vi "Main Editor UI.vi"() -> ()   [LabVIEW 2015, in "DAQmx Module editor node.lvclass"]
doc: "This is the main view for configuration the behavior of a module in the DCAF standard editor."
uses:
  DAQmx Module editor node.lvclass
  <vilib>/NI/Configuration Framework/Node/NodeRef.ctl
  <vilib>/NI/Configuration Framework/Node/NISE_CEF_Node.lvclass
  <vilib>/NI/AMC/Message Queue.ctl
  <vilib>/NI/AMC/Message.ctl
  <vilib>/NI/Tools/Keyed Array/KeyedArray.ctl
  <vilib>/NI/Configuration Framework/Node/UserEventRef.ctl
  <vilib>/NI/Configuration Framework/Controls/EventCluster.ctl
  <vilib>/NI/DCAF UI Toolkit/Controls/Configure.ctl
  <vilib>/NI/DCAF UI Toolkit/Controls/Add.ctl
  <vilib>/NI/DCAF UI Toolkit/Controls/Remove.ctl
  <vilib>/NI/Configuration Framework/Node/StopEvent.ctl
  <vilib>/NI/Configuration Framework/Node/RefreshUIEvent.ctl
  <vilib>/NI/Configuration Framework/Node/CacheState.ctl
  <vilib>/NI/Configuration Framework/Node/NodeChangeEvent.ctl
  <vilib>/NI/DCAF/Tag Editor Core/Table API/Available Tag Menu/channel action event.ctl
  <vilib>/NI/DCAF/Tag Editor Core/Table API/Available Tag Menu/dialog output action.ctl
  <vilib>/NI/Tag Bus Module Framework/channel/TBM channel.lvclass
  <vilib>/NI/Tag Bus/tag/tag descriptor.lvclass
  <vilib>/NI/DCAF/Tag Editor Core/Table API/Table Manager/Call Back Ref Type Def.ctl
  <vilib>/NI/DCAF/Tag Editor Core/Configuration Editor/Classes/Engine Parent/Engine Parent Editor Node.lvclass
  <vilib>/NI/DCAF/Tag Editor Core/Configuration Editor/Classes/Module editor node/module editor node.lvclass
  <vilib>/NI/DCAF UI Toolkit/Controls/Import.ctl
  <vilib>/NI/DCAF UI Toolkit/Controls/Export.ctl
  <vilib>/NI/DCAF/Tag Editor Core/Table API/Table Manager/references.ctl
  module/configuration/Daqmx Module configuration.lvclass/Daqmx Module configuration.ctl
  <vilib>/Utility/miscctls.llb/LVPositionTypeDef.ctl
  <vilib>/NI/DCAF/Tag Editor Core/Table API/Listbox/Multi Column Listbox.lvclass
  <vilib>/NI/Configuration Framework/NISE_CEF_TreeControl.lvlib
  <vilib>/NI/Tools/Keyed Array/Tools_KeyedArray.lvlib
  <vilib>/NI/AMC/AMC.lvlib
  <vilib>/NI/DCAF/Tag Editor Core/Table API/Table Manager.lvlib
  <vilib>/NI/DCAF/Tag Editor Core/Table API/Table Manager/Table Manager.lvclass
  <vilib>/NI/DCAF UI Toolkit/Controls/DCAF UI Elements.lvlib
  module/configuration/Daqmx Module configuration.lvclass
panel:
  in  "user event out":refnum<user-event>
  in  "node change":T1
  in  "cache state":T2
  in  "refresh UI":T3
  in  "stop event":T4
  in  "Tab Control":T5(tab)
  in  "Remove Button":T6
  in  "Add Button":T7
  in  "Table":i32(listbox)
  in  "settings":T8
  in  "Export":T9
  in  "Import":T10
  in  "Data Rate (Hz)":dbl=1.0 min=1.0 step=1.0
  in  "user event":T11
  in  "main queue":T12
  in  "node ref":T13
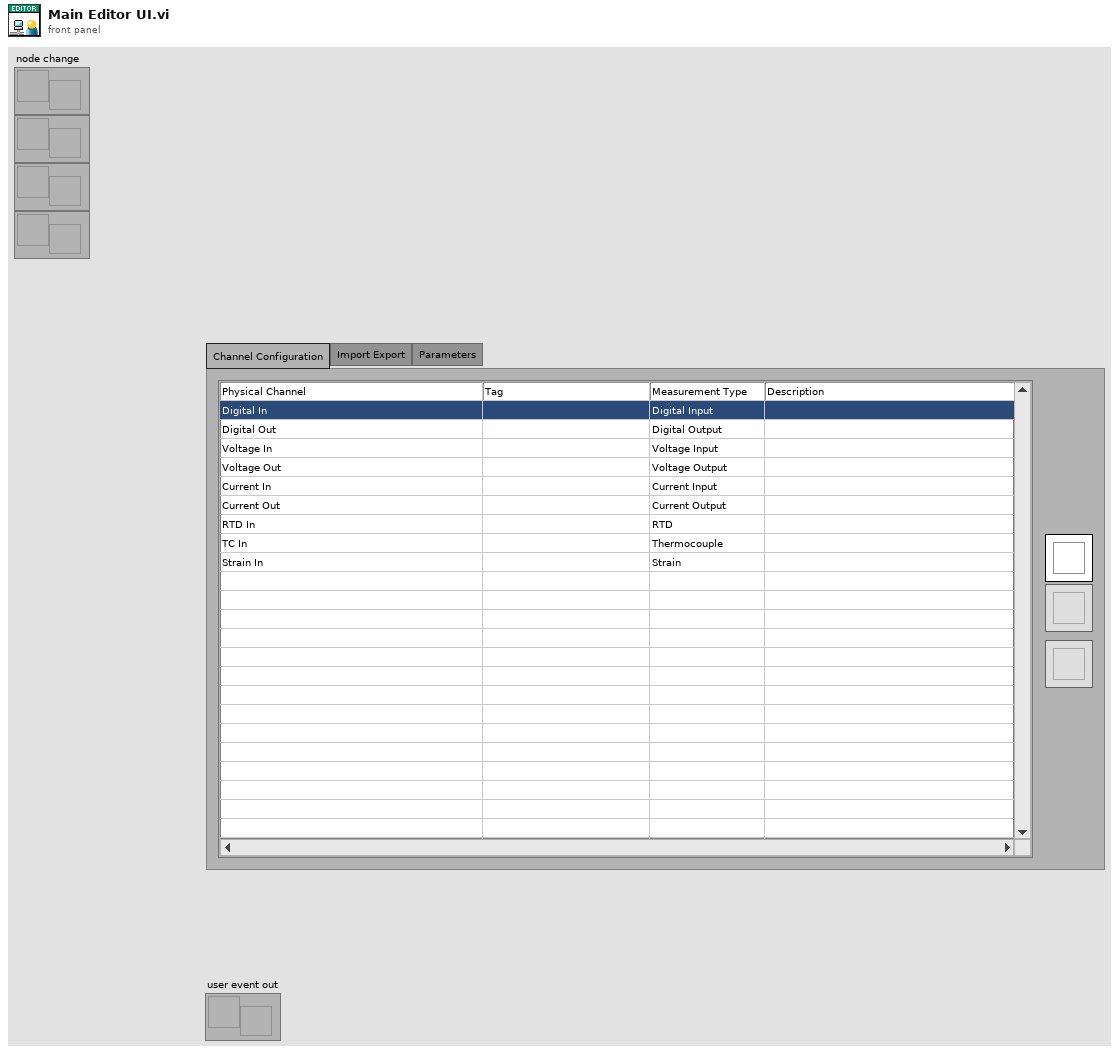
[diagram p1: front panel]
types:
  T1 = typedef "NISE_CEF_Node.lvclass/NodeChangeEvent.ctl" = refnum<user-event>
  T2 = typedef "NISE_CEF_Node.lvclass/CacheState.ctl" = refnum<user-event>
  T3 = typedef "NISE_CEF_Node.lvclass/RefreshUIEvent.ctl" = refnum<user-event>
  T4 = typedef "NISE_CEF_Node.lvclass/StopEvent.ctl" = refnum<user-event>
  T5 = enum32{"Channel Configuration", "Import Export", "Parameters"}
  T6 = typedef "DCAF UI Elements.lvlib/Remove.ctl" = bool
  T7 = typedef "DCAF UI Elements.lvlib/Add.ctl" = bool
  T8 = typedef "DCAF UI Elements.lvlib/Configure.ctl" = bool
  T9 = typedef "DCAF UI Elements.lvlib/Export.ctl" = bool
  T10 = typedef "DCAF UI Elements.lvlib/Import.ctl" = bool
  T11 = typedef "NISE_CEF_Node.lvclass/UserEventRef.ctl" = refnum<user-event>
  T12 = typedef "AMC.lvlib/Message Queue.ctl" = refnum<queue>
  T13 = typedef "NISE_CEF_Node.lvclass/NodeRef.ctl" = refnum<data-value>
  T14 = typedef "Table Manager.lvlib/Table Manager.lvclass/references.ctl" = cluster{"stop event":T4, "refresh UI":T3, "cache state":T2, "node change":T1, "user event out":refnum<user-event>, "main queue":T12, "user event":T11}
  T15 = typedef "LVPositionTypeDef.ctl" = cluster{"Left":i32, "Top":i32}
  T16 = typedef "Table Manager.lvlib/Table Manager.lvclass/object ref.ctl" = cluster{"engine":refnum<data-value>, "Node Ref":refnum<data-value>}
  T17 = typedef "Table Manager.lvlib/Column.lvclass/Column Descriptor.ctl" = cluster{"name":string, "caption":string, "Column Type":T18, "Params":string, "AutoSizeMode":i32, "FillWeight":sgl, "MinWidth":u32, "tooltip":string, "Enum Reference":refnum<vi>, "Channel suffix":string, "Read Only":bool, "Call Back VI":T19, "DT Dependency":i32, "name dependency":i32, "data type":T20, "Custom Column":refnum<class "Column.lvclass">}
  T18 = typedef "Table Manager.lvlib/Column.lvclass/Column Type.ctl" = enum16{"String", "Mapping", "Enum", "Custom"}
  T19 = typedef "Table Manager.lvlib/Table Manager.lvclass/Call Back Ref Type Def.ctl" = refnum<vi>
  T20 = typedef "tag bus.lvlib/tag descriptor.lvclass/Data Type.ctl" = enum16{"Double", "Single", "I64", "I32", "I16", "I8", "U64", "U32", "U16", "U8", "Boolean", "String", "Array of Double", "Array of Single", "Array of I64", "Array of I32", "Array of I16", "Array of I8", "Array of U64", "Array of U32", "Array of U16", "Array of U8", "Array of Boolean", "Array of String"}
  T21 = typedef "Table Manager.lvlib/Table Manager.lvclass/Table Events.ctl" = cluster{"Menu Selection":refnum<user-event>}
  T22 = enum8{"Enabled", "Disabled", "Disabled and Grayed Out"}
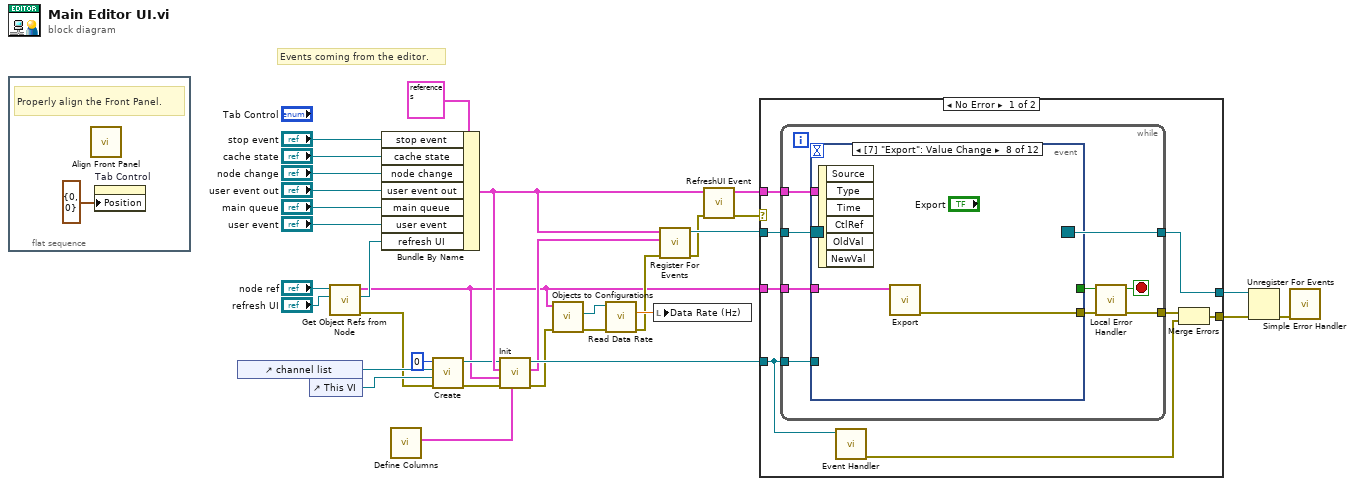
[diagram p0: block diagram]
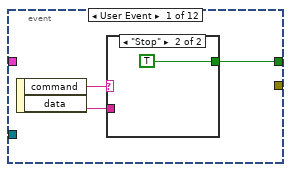
[diagram p2: hidden frame]
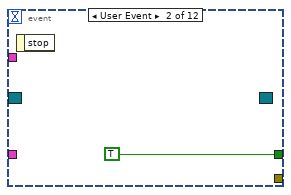
[diagram p4: hidden frame]
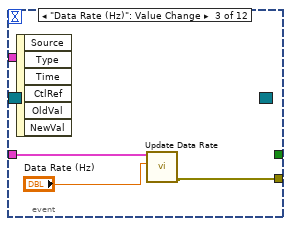
[diagram p5: hidden frame]
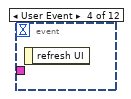
[diagram p6: hidden frame]
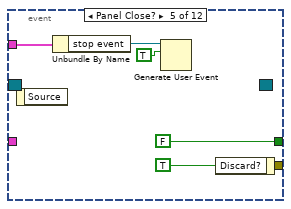
[diagram p7: hidden frame]
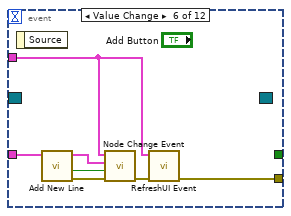
[diagram p8: hidden frame]
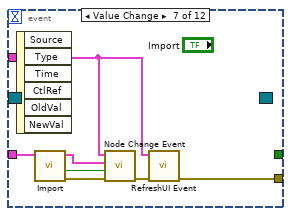
[diagram p9: hidden frame]
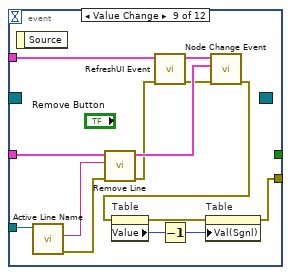
[diagram p10: hidden frame]
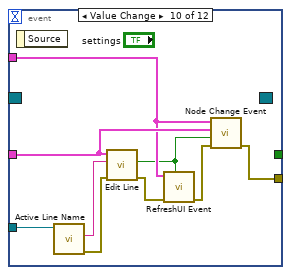
[diagram p11: hidden frame]
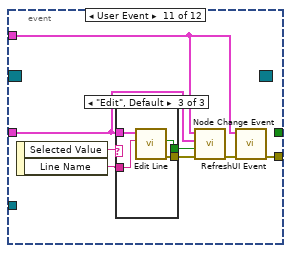
[diagram p12: hidden frame]
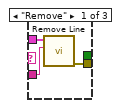
[diagram p13: hidden frame]
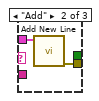
[diagram p14: hidden frame]
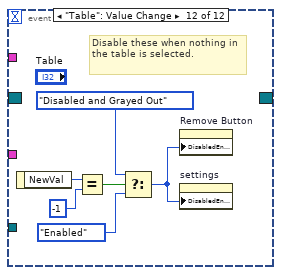
[diagram p15: hidden frame]
diagram:
  # "Events coming from the editor."
  n1 = flat-sequence {
    frame #0 {
      # "Properly align the Front Panel."
      n2 = call <vilib>:"Align Front Panel.vi"() -> ()  [unwired: 10 in, 2 out]
      n3 = property on="Tab Control" class="TabCtl (strict)"("Position"=T15 {"Left"=0, "Top"=0}) -> ()  [unwired: 2 in, 2 out]
    }
  }
  n4 = control-ref of="channel list"() -> (w14:refnum<vi>)
  n5 = control-ref of="This VI"() -> (w12:refnum<vi>)
  n6 = call "Get Object Refs from Node.vi"("Refresh UI"="refresh UI", "Data Value Reference in"="node ref") -> ("error out"=w9:errorcluster, "Refresh UI out"=w7:T3, "References"=w1:T16)  [unwired: 7 in]
  n7 = Bundle By Name(cluster=T14 {"stop event"=refnum, "refresh UI"=refnum, "cache state"=refnum, "node change"=refnum, "user event out"=refnum, "main queue"=refnum, "user event"=refnum} ("References"), "stop event"="stop event", "cache state"="cache state", "node change"="node change", "user event out"="user event out", "main queue"="main queue", "user event"="user event", "refresh UI"=w7) -> (w20:T14)
  n8 = call "Define Columns.vi"() -> ("Column Definition"=w22:T17[])  [unwired: 11 in]
  n9 = call <vilib>:"Create.vi"("error in (no error)"=w9, "Top VI"=w12, "Listbox"=w14, "Index"=0) -> ("error out"=w10:errorcluster, "reference out"=w11:refnum<class "Multi Column Listbox.lvclass">)  [unwired: 6 in]
  n10 = call-dynamic "Init.vi"("Column Descriptors"=w22, "error in (no error)"=w10, "Node object refs"=w1, "Event References"=w20, "Multi Column Listbox in"=w11) -> ("error out"=w4:errorcluster, "Table Events"=w15:T21, "Multi Column Listbox out"=w19:refnum<class "Multi Column Listbox.lvclass">)  [unwired: 4 in]
  n11 = call "Objects to Configurations.vi"("error in (no error)"=w4, "Objects in"=w1) -> ("error out"=w5:errorcluster, "tag bus configurable plugin module configuration"=w6:refnum<class "Daqmx Module configuration.lvclass">)  [unwired: 7 in, 1 out]
  n12 = call "Read Data Rate.vi"("error in (no error)"=w5, "Daqmx Module configuration in"=w6) -> ("error out"=w2:errorcluster, "Rate"=w3:dbl)  [unwired: 7 in, 1 out]
  n13 = local write "Data Rate (Hz)"(w3) -> ()
  n14 = call "Register For Events.vi"("error in"=w2, "Table Events"=w15, "References"=w20) -> ("error out"=w17:errorcluster, "Event Registration Refnum"=w23:refnum<event-registration>)  [unwired: 7 in]
  n15 = call "RefreshUI Event.vi"("error in (no error)"=w17, "References in"=w20) -> ("error out"=w16:errorcluster, "References out"=w21:T14)  [unwired: 8 in]
  n16 = case shown="No Error" w16 {
    selector: w16 -> [_ w126]
    tunnel: w23 -> [w42 w125]
    tunnel: [w41 w125] -> w33
    tunnel: [w35 w126] -> w32
    tunnel: w21 -> [w40 _]
    tunnel: w1 -> [w39 _]
    tunnel: w19 -> [w38 _]
    frame No Error {
      n17 = while {
        tunnel: w42 -> [w51]
        tunnel: [w50] -> w41
        tunnel: [w47] -> w36
        tunnel: w40 -> [w45]
        tunnel: w39 -> [w44]
        tunnel: w38 -> [w43]
        stop <- w49 stop-if-true
        n18 = event shown="[7] \"Export\": Value Change" {
          selector: w51 -> [_ _ _ _ _ _ _ _ _ _ _ _]
          dyn-events: [_ _ _ _ _ _ _ _ _ _ _ _] -> w50
          timeout: _ -> [_ _ _ _ _ _ _ _ _ _ _ _]
          tunnel: [w54 TRUE _ _ FALSE _ _ _ _ _ _ _] -> w48
          tunnel: [_ _ w58 _ _ w65 w75 w78 w81 w101 w107 _] -> w46
          tunnel: w45 -> [_ _ _ _ w61 w69 w77 _ w92 w96 w103 _]
          tunnel: w44 -> [_ _ w59 _ _ w70 w72 w79 w91 w99 w104 _]
          tunnel: w43 -> [_ _ _ _ _ _ _ _ w87 w100 _ _]
          event User Event {
            n19 = event-data() -> ("command"=w53:string, "data"=w52:string)  [unwired: 1 in]
            n20 = case shown="\"Stop\"" w53 {
              tunnel: [_ TRUE] -> w54
              tunnel: w52 -> [_ _]
              frame Default {
              }
              frame "Stop" {
              }
            }
          }
          event User Event {
            n21 = event-data() -> ()  [unwired: 1 in, 1 out]
          }
          event "Data Rate (Hz)": Value Change {
            n22 = event-data() -> ()  [unwired: 1 in, 6 out]
            n23 = call "Update Data Rate.vi"("Rate"="Data Rate (Hz)", "objects"=w59) -> ("error out"=w58:errorcluster)  [unwired: 9 in]
          }
          event User Event {
            n24 = event-data() -> ()  [unwired: 1 in, 1 out]
          }
          event Panel Close? {
            n25 = event-data() -> ()  [unwired: 1 in, 1 out]
            n26 = Unbundle By Name(w61) -> ("stop event"=w60:T4)
            n27 = Generate User Event(user event=w60, event data cluster=TRUE ("event data")) -> ()  [unwired: 2 in, 2 out]
            n28 = event-data("Discard?"=TRUE) -> ()  [unwired: 1 in, 1 out]
          }
          event Value Change {
            n29 = event-data() -> ()  [unwired: 1 in, 1 out]
            n30 = call "Add New Line.vi"("objects"=w70) -> ("error out"=w68:errorcluster, "success"=w66:bool)  [unwired: 8 in, 1 out]
            n31 = call "Node Change Event.vi"("error in (no error)"=w68, "Send (T)"=w66, "objects"=w70, "References in"=w69) -> ("error out"=w67:errorcluster)  [unwired: 7 in]
            n32 = call "RefreshUI Event.vi"("error in (no error)"=w67, "References in"=w69) -> ("error out"=w65:errorcluster)  [unwired: 8 in, 1 out]
          }
          event Value Change {
            n33 = event-data() -> ()  [unwired: 1 in, 6 out]
            n34 = call "Import.vi"("Objects in"=w72) -> ("error out"=w74:errorcluster, "Update"=w73:bool, "Objects out"=w71:T16)  [unwired: 8 in]
            n35 = call "Node Change Event.vi"("error in (no error)"=w74, "Send (T)"=w73, "objects"=w71, "References in"=w77) -> ("error out"=w76:errorcluster)  [unwired: 7 in]
            n36 = call "RefreshUI Event.vi"("error in (no error)"=w76, "References in"=w77) -> ("error out"=w75:errorcluster)  [unwired: 8 in, 1 out]
          }
          event Value Change {
            n37 = event-data() -> ()  [unwired: 1 in, 6 out]
            n38 = call "Export.vi"("Objects"=w79) -> ("error out"=w78:errorcluster)  [unwired: 10 in]
          }
          event Value Change {
            n39 = event-data() -> ()  [unwired: 1 in, 1 out]
            n40 = call-dynamic "Active Line Name.vi"("Multi Column Listbox in"=w87) -> ("error out"=w85:errorcluster, "Active Line Name"=w86:string)  [unwired: 8 in, 1 out]
            n41 = call "Remove Line.vi"("error in"=w85, "Active Line Name"=w86, "Objects"=w91) -> ("error out"=w88:errorcluster)  [unwired: 8 in]
            n42 = call "RefreshUI Event.vi"("error in (no error)"=w88, "References in"=w92) -> ("error out"=w90:errorcluster, "References out"=w89:T14)  [unwired: 8 in]
            n43 = call "Node Change Event.vi"("error in (no error)"=w90, "objects"=w91, "References in"=w89) -> ("error out"=w82:errorcluster)  [unwired: 8 in]
            n44 = property on="Table" class="MCListbox (strict)"(error in=w82) -> (error out=w80:errorcluster, "Value"=w83:i32)  [unwired: 1 in, 1 out]
            n45 = Decrement(x=w83) -> (x-1=w84:i32)
            n46 = property on="Table" class="MCListbox (strict)"(error in=w80, "Val(Sgnl)"=w84) -> (error out=w81:errorcluster)  [unwired: 1 in, 1 out]
          }
          event Value Change {
            n47 = event-data() -> ()  [unwired: 1 in, 1 out]
            n48 = call-dynamic "Active Line Name.vi"("Multi Column Listbox in"=w100) -> ("error out"=w97:errorcluster, "Active Line Name"=w98:string)  [unwired: 8 in, 1 out]
            n49 = call "Edit Line.vi"("error in"=w97, "Line Name"=w98, "References"=w99) -> ("error out"=w94:errorcluster, "change?"=w95:bool)  [unwired: 7 in]
            n50 = call "RefreshUI Event.vi"("Refresh (T)"=w95, "error in (no error)"=w94, "References in"=w96) -> ("error out"=w93:errorcluster)  [unwired: 7 in, 1 out]
            n51 = call "Node Change Event.vi"("error in (no error)"=w93, "Send (T)"=w95, "objects"=w99, "References in"=w96) -> ("error out"=w101:errorcluster)  [unwired: 7 in]
          }
          event User Event {
            n52 = event-data() -> ("Selected Value"=w109:string, "Line Name"=w106:string)  [unwired: 1 in]
            n53 = case shown="\"Edit\", Default" w109 {
              tunnel: w106 -> [w112 _ w118]
              tunnel: w104 -> [w111 w114 w117]
              tunnel: [w110 w113 w116] -> w105
              tunnel: [_ _ w115] -> w102
              frame "Remove" {
                n54 = call "Remove Line.vi"("Active Line Name"=w112, "Objects"=w111) -> ("error out"=w110:errorcluster)  [unwired: 9 in]
              }
              frame "Add" {
                n55 = call "Add New Line.vi"("objects"=w114) -> ("error out"=w113:errorcluster)  [unwired: 8 in, 2 out]
              }
              frame "Edit", Default {
                n56 = call "Edit Line.vi"("Line Name"=w118, "References"=w117) -> ("error out"=w116:errorcluster, "change?"=w115:bool)  [unwired: 8 in]
              }
            }
            n57 = call "Node Change Event.vi"("error in (no error)"=w105, "Send (T)"=w102, "objects"=w104, "References in"=w103) -> ("error out"=w108:errorcluster)  [unwired: 7 in]
            n58 = call "RefreshUI Event.vi"("error in (no error)"=w108, "References in"=w103) -> ("error out"=w107:errorcluster)  [unwired: 8 in, 1 out]
          }
          event "Table": Value Change {
            # "Disable these when nothing in the table is selected."
            n59 = event-data() -> ("NewVal"=w124:i32)  [unwired: 1 in]
            n60 = Equal?(x=w124, y=-1) -> (x = y?=w122:bool)
            n61 = Select(t=T22."Disabled and Grayed Out" ("Disabled"), s=w122, f=T22."Enabled") -> (s? t:f=w120:T22)
            n62 = property on="Remove Button" class="Bool"("DisabledEnum"=w120) -> ()  [unwired: 2 in, 2 out]
            n63 = property on="settings" class="Bool"("DisabledEnum"=w120) -> ()  [unwired: 2 in, 2 out]
          }
        }
        n64 = call "Local Error Handler.vi"("error in"=w46, "Stop in"=w48) -> ("error out"=w47:errorcluster, "Stop out"=w49:bool)  [unwired: 8 in]
      }
      n65 = call-dynamic "Event Handler.vi"("Listbox in"=w38) -> ("error out"=w37:errorcluster)  [unwired: 9 in, 1 out]
      n66 = Merge Errors(w36, w37) -> (w35:errorcluster)
    }
    frame Error {
    }
  }
  n67 = Unregister For Events(event registration refnum=w33, error in=w32) -> (error out=w31:errorcluster)
  n68 = call <vilib>:"Simple Error Handler.vi"("error in (no error)"=w31) -> ()  [unwired: 4 in, 5 out]
